vi "errorDebug.vi"() -> ()   [LabVIEW 2013]
panel:
  in  "Error Code":dbl
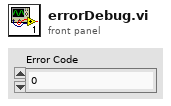
[diagram p1: front panel]
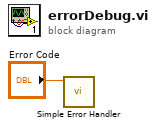
[diagram p0: block diagram]
diagram:
  n1 = call <vilib>:"Simple Error Handler.vi"("error code (no error:0)"="Error Code") -> ()  [unwired: 4 in, 5 out]
